vi "ImPro - UI Text.vi"(7 "Directory Path":path, 8 "error in (no error)":errorcluster, 10 "Supervisory Config Cluster Out":T3={"UI Information"={"Header Image"=path "../Data/header.png", "Language"=enum."English", "First Run?"=FALSE, "Setup Camera?"=FALSE, "Device Type"=enum."RCA", "Encoder Type"=enum."Tacho", "Version"=enum."RailMeasurement_CAT", "port"=0, "greyscale"=FALSE, "camera index"=0}, "Test Cluster"={"Operator"="", "Description"="", "Line"="", "Start Position"=450000.0, "Run Length"=31.0, "Sensor A Position"=80000.0, "Rail Side"=FALSE, "Distance Direction"=FALSE, "Path"=path "", "Sensor B Position"=0.0, "Visible Chart Distance"=0.0, "Company"="", "Ref Profile"=""}, "RV-HR Settings Cluster"={"Sensor A Calibration"=0.0, "Integrator Time"=0.0, "Encoder Spacing"=0.0, "Encoder Threshold"=0.0, "Sampling Distance"=0, "Swap Direction?"=FALSE, "Min Walking Speed"=0.0, "Max Walking Speed"=0.0, "Distance Format"=0, "Sensor B Calibration"=0.0, "Tacho Pulses/Rev"=0.0, "Wheel Diameter"=0.0, "Max Short Roughness"=0.0, "Max Long Roughness"=0.0, "Measuring Interval"=0.0, "Measuring Length"=0.0, "Wavelengths"=[], "Device Resolution"=0, "Detect Change in Direction?"=FALSE, "Save Images?"=FALSE, "Image Frequency"=0, "Save Video?"=FALSE, "Image Offset"=0.0, "Start Position at 0m?"=FALSE, "Live Corrug Est.?"=FALSE, "Wavelength Corrug"=0, "Distance Corrug"=0, "Update Corrug"=0}} {"RV-HR Settings Cluster"."Image Frequency" items=["2", "3", "5"]; "RV-HR Settings Cluster"."Device Resolution" items=["0.1 µm", "1 µm", "10 µm"]; "RV-HR Settings Cluster"."Distance Format" items=["kilometres", "miles & chains", "metres", "stations", "miles"]; "RV-HR Settings Cluster"."Sampling Distance" items=["1mm", "2mm"]}, 11 "UI References":T13) -> (0 "error out":errorcluster, 1 "UI Information.Language":T1, 2 "Language Config Cluster Out":T2={"Home"="Home", "Test Setup"="Setup", "Run Test"="Test", "Configure"="Config", "Hardware Viewer"="Viewer", "Review Test"="Review", "Report"="Home", "Exit"="Exit", "Device Connected?"="Device Connected?", "Test in Progress?"="Test in Progress?", "Simulate?"="Simulate?", "Device Type 1"="Corrugation Analysis Trolley", "Device Type 2"="Bi-Corrugation Analysis Trolley", "Device Type 3"="Bi-Corrugation Analysis Trolley", "Device Type 4"="Bi-Corrugation Analysis Trolley", "Device Type 5"="Bi-Corrugation Analysis Trolley", "Device Type 6"="Bi-Corrugation Analysis Trolley", "Device Type 7"="Bi-Corrugation Analysis Trolley", "Software Version"="Version", "Support"="Software by RailMeasurement Limited - Cambridge - UK - support@railmeasurement.com", "Operator"="Operator:", "Test Description"="Description:", "Line"="Description:", "Test Folder Path"="Folder Path:", "Test Folder Path RCA"="Folder Path:", "Start Position"="Start Position:", "Sensor Position"="Sensor Position:", "Sensor A Position"="Sensor A Position:", "Sensor B Position"="Sensor B Position:", "Visible Chart Distance"="Sensor B Position:", "Rail Side"="Rail Side:", "Rail A Side"="Rail A Side:", "Distance Direction"="Distance Direction:", "Start"="Start:", "Distance Travelled"="Distance Travelled:", "Current Position"="Current Position:", "Stop Test"="Stop", "Pause Test"="Save", "Displacement"="Displacement", "Position"="Position", "Sensor Calibration"="Sensor Calibration:", "Sensor A Calibration"="Sensor A Calibration:", "Sensor B Calibration"="Sensor B Calibration:", "Encoder Spacing"="Encoder Spacing:", "Sampling Distance"="Sampling Distance:", "Tacho Pulses/Rev"="Sensor Calibration:", "Wheel Diameter"="Sensor A Calibration:", "Sampling Distances"=["1mm", "2mm"], "Distance Unit"="Distance in:", "Distance Units"=["Kilometres", "miles & chains", "metres", "stations", "miles"], "Swap Direction"="Swap Direction at Run End?", "Language"="Language", "Device Resolution"="Save", "Device Resolutions"=["Kilometres", "miles & chains", "metres", "stations", "miles"], "Detect Change in Direction"="Save", "Save Config"="Save", "Encoder Data"="Encoder Data", "Sensor Data"="Sensor Data", "Sensor A Data"="Sensor A Data", "Sensor B Data"="Sensor B Data", "Voltage"="Voltage", "Time (m:s)"="Time (m:s)", "Unit mm/s/V"="(mm/s)/V", "Unit mm"="mm", "Unit km"="km", "Unit m"="m", "Start Test Message"="m", "Stop Test Message"="km", "Exit Message"="mm", "File Exists Message"="mm", "File Path Invalid Message"="mm", "Combine Error"="mm", "Combine Success"="mm", "Roller Comp Error"="mm", "Test Folder Path (Live)"="mm", "Folder Error"="Sensor B Position:", "Enc Count"="Setup", "Run Start"="mm", "Run End"="mm", "Date"="mm", "Train"="Sensor B Position:", "Location"="Setup", "Notes"="mm", "Heading_1"="mm", "Heading_2"="mm", "Left Rail"="Sensor B Position:", "Right Rail"="Setup", "Left Exclusions"="mm", "Right Exclusions"="mm", "Settings"="mm", "Wavelength Ranges"="Sensor B Position:", "Y-Axis Limits"="Setup", "Exc Limits"="Sensor B Position:", "Other Settings"="Setup", "Distance/Page"="mm", "Distance/Pages"=["Kilometres", "miles & chains", "metres", "stations", "miles"], "Gridlines"="mm", "Report Tolerance"="mm", "Manual Cut"="Sensor B Position:", "Plot Colour"="Distance in:", "Plot Colours"=["Kilometres", "miles & chains", "metres", "stations", "miles"], "EN Standard"="mm", "RiL Standard"="mm", "Custom Standard"="mm", "Resolution"="Distance in:", "Resolutions"=["Kilometres", "miles & chains", "metres", "stations", "miles"], "Exceedence Header"="mm", "Distance (km)"="mm", "Left (%)"="mm", "Right (%)"="Distance in:", "Page"="Distance in:", "Align"="mm", "Main"="mm", "Comparison"="Distance in:", "Offset"="Distance in:", "From"="Distance in:", "To"="Distance in:", "Of"="Distance in:", "File"="mm", "Load New"="mm", "Load Comparison"="Distance in:", "Discard Comparison"="Distance in:", "Print Current Page"="Distance in:", "Print All Pages"="Distance in:", "Print Exceedence Report"="Distance in:", "Plot Main"="Distance in:", "No Comparison Data to Align"="Distance in:", "Run Load Error"="Distance in:", "Report Load Error"="Distance in:", "Cut"="Distance in:", "Remove"="Distance in:", "Config Settings Unsaved"="Distance in:", "Acquisition Paused"="Distance in:", "Please Select One Option Below"="Distance in:", "RCA is Now Stationary"="Distance in:", "Reporting Setting"="Distance in:", "Main Abbreviated"="Distance in:", "Comparison Abbreviated"="Distance in:", "Exceedence Abbreviated"="Distance in:", "Align Comparison"="Distance in:", "Rail Corrugation Analyser Reporting"="Distance in:", "Show Exc. % in Graph"="Distance in:", "Evaluate Sections <100m"="Distance in:", "Evaluate Sections <0.062mile"="Distance in:", "Section Too Short for Evaluation"="Distance in:", "Language Change Prompt"="Distance in:", "Show All"="Distance in:", "Sections_km"="Distance in:", "Sections_mi"="Distance in:", "Vision"="Distance in:", "Vision Report"="Distance in:", "Vision Display"="Distance in:", "Vision Displays"=["Kilometres", "miles & chains", "metres", "stations", "miles"], "Save Images"="Distance in:", "Image Frequency"="Distance in:", "Section"="Distance in:", "Brightness"="Distance in:", "Contrast"="Distance in:", "Shadow"="Distance in:", "Sharpened"="Distance in:", "Apply to all Images"="Distance in:", "Reset"="Distance in:", "Are you sure"="Distance in:", "Image Processing"="Distance in:", "Save Video"="Distance in:", "Image Offset"="Distance in:", "Camera Mode"="Distance in:", "Camera Modes"=["Kilometres", "miles & chains", "metres", "stations", "miles"], "Copy Page"="Distance in:", "Copy Graphs"="Distance in:", "Camera Mode Change Prompt"="Distance in:", "Camera_1 Missing"="Distance in:", "Camera_2 Missing"="Distance in:", "Cameras Missing"="Distance in:", "Camera Setup"="Distance in:", "Camera_1 Connection Error"="Distance in:", "Camera_2 Connection Error"="Distance in:", "Cameras Connection Error"="Distance in:", "No GPS"="Distance in:", "No Signal"="Distance in:", "Camera_1 Connected"="Distance in:", "Camera_1 Not Connected"="Distance in:", "Camera_2 Connected"="Distance in:", "Camera_2 Not Connected"="Distance in:", "Start Position at 0m?"="Distance in:", "Continue"="Distance in:", "New Test, Same Direction"="Distance in:", "New Test, Opposite Direction"="Distance in:", "Stop and Save"="Distance in:", "Live Corrug Estimate"="Distance in:", "Wavelength Corrug"="Distance in:", "Distance Corrug "="Distance in:", "Update Corrug"="Distance in:", "Company"="Distance in:", "Ref Profile "="Distance in:"}, 3 "Support":string)   [LabVIEW 2023]
uses:
  Controls/Language.ctl
  <vilib>/addons/Tools/Unicode/UI Unicode Tools.lvlib
  Controls/Device_Type.ctl
  Controls/UI Init Config Info.ctl
  Controls/Test Cluster.ctl
  Controls/Sampling DIstance.ctl
  Controls/Distance Units.ctl
  Controls/Settings Cluster.ctl
  Controls/Supervisory Config Cluster.ctl
  Controls/Language Text Cluster.ctl
  Controls/EncoderType.ctl
  Controls/Device_Resolution.ctl
  Controls/Software Version.ctl
  Controls/ImPro - UI Refs.ctl
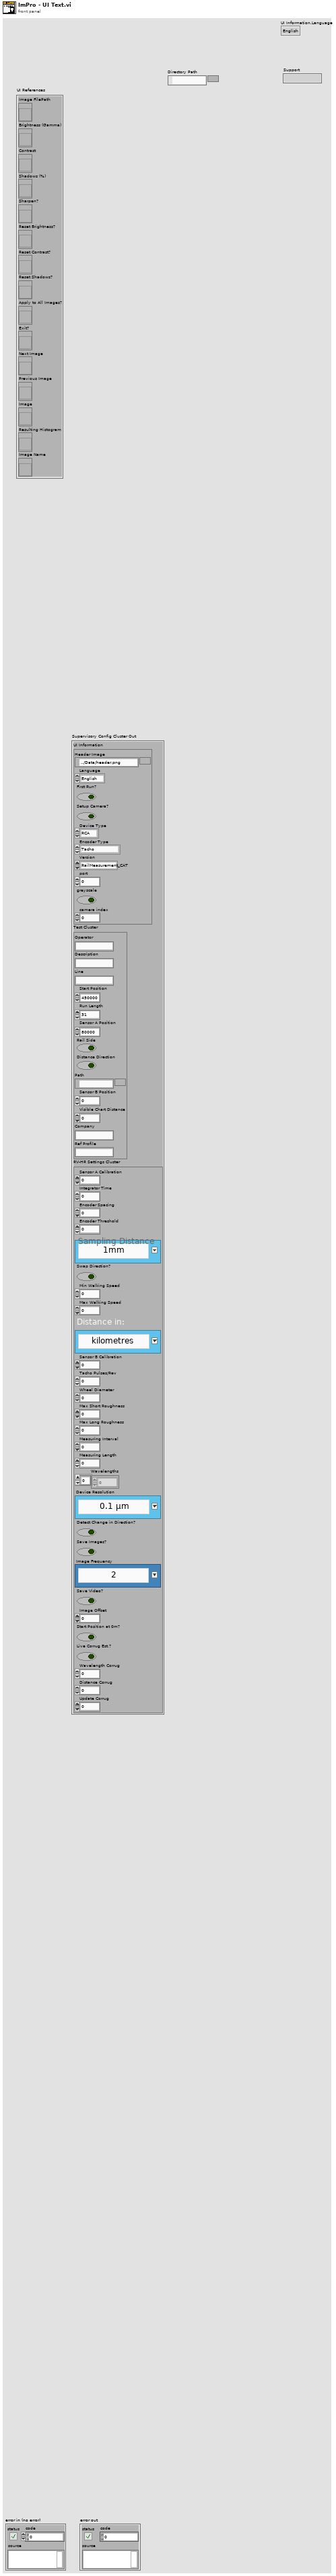
[diagram p1: front panel]
types:
  T1 = typedef "Language.ctl" = enum16{"English", "Chinese", "German"}
  T2 = typedef "Language Text Cluster.ctl" = cluster{"Home":string, "Test Setup":string, "Run Test":string, "Configure":string, "Hardware Viewer":string, "Review Test":string, "Report":string, "Exit":string, "Device Connected?":string, "Test in Progress?":string, "Simulate?":string, "Device Type 1":string, "Device Type 2":string, "Device Type 3":string, "Device Type 4":string, "Device Type 5":string, "Device Type 6":string, "Device Type 7":string, "Software Version":string, "Support":string, "Operator":string, "Test Description":string, "Line":string, "Test Folder Path":string, "Test Folder Path RCA":string, "Start Position":string, "Sensor Position":string, "Sensor A Position":string, "Sensor B Position":string, "Visible Chart Distance":string, "Rail Side":string, "Rail A Side":string, "Distance Direction":string, "Start":string, "Distance Travelled":string, "Current Position":string, "Stop Test":string, "Pause Test":string, "Displacement":string, "Position":string, "Sensor Calibration":string, "Sensor A Calibration":string, "Sensor B Calibration":string, "Encoder Spacing":string, "Sampling Distance":string, "Tacho Pulses/Rev":string, "Wheel Diameter":string, "Sampling Distances":string[], "Distance Unit":string, "Distance Units":string[], "Swap Direction":string, "Language":string, "Device Resolution":string, "Device Resolutions":string[], "Detect Change in Direction":string, "Save Config":string, "Encoder Data":string, "Sensor Data":string, "Sensor A Data":string, "Sensor B Data":string, "Voltage":string, "Time (m:s)":string, "Unit mm/s/V":string, "Unit mm":string, "Unit km":string, "Unit m":string, "Start Test Message":string, "Stop Test Message":string, "Exit Message":string, "File Exists Message":string, "File Path Invalid Message":string, "Combine Error":string, "Combine Success":string, "Roller Comp Error":string, "Test Folder Path (Live)":string, "Folder Error":string, "Enc Count":string, "Run Start":string, "Run End":string, "Date":string, "Train":string, "Location":string, "Notes":string, "Heading_1":string, "Heading_2":string, "Left Rail":string, "Right Rail":string, "Left Exclusions":string, "Right Exclusions":string, "Settings":string, "Wavelength Ranges":string, "Y-Axis Limits":string, "Exc Limits":string, "Other Settings":string, "Distance/Page":string, "Distance/Pages":string[], "Gridlines":string, "Report Tolerance":string, "Manual Cut":string, "Plot Colour":string, "Plot Colours":string[], "EN Standard":string, "RiL Standard":string, "Custom Standard":string, "Resolution":string, "Resolutions":string[], "Exceedence Header":string, "Distance (km)":string, "Left (%)":string, "Right (%)":string, "Page":string, "Align":string, "Main":string, "Comparison":string, "Offset":string, "From":string, "To":string, "Of":string, "File":string, "Load New":string, "Load Comparison":string, "Discard Comparison":string, "Print Current Page":string, "Print All Pages":string, "Print Exceedence Report":string, "Plot Main":string, "No Comparison Data to Align":string, "Run Load Error":string, "Report Load Error":string, "Cut":string, "Remove":string, "Config Settings Unsaved":string, "Acquisition Paused":string, "Please Select One Option Below":string, "RCA is Now Stationary":string, "Reporting Setting":string, "Main Abbreviated":string, "Comparison Abbreviated":string, "Exceedence Abbreviated":string, "Align Comparison":string, "Rail Corrugation Analyser Reporting":string, "Show Exc. % in Graph":string, "Evaluate Sections <100m":string, "Evaluate Sections <0.062mile":string, "Section Too Short for Evaluation":string, "Language Change Prompt":string, "Show All":string, "Sections_km":string, "Sections_mi":string, "Vision":string, "Vision Report":string, "Vision Display":string, "Vision Displays":string[], "Save Images":string, "Image Frequency":string, "Section":string, "Brightness":string, "Contrast":string, "Shadow":string, "Sharpened":string, "Apply to all Images":string, "Reset":string, "Are you sure":string, "Image Processing":string, "Save Video":string, "Image Offset":string, "Camera Mode":string, "Camera Modes":string[], "Copy Page":string, "Copy Graphs":string, "Camera Mode Change Prompt":string, "Camera_1 Missing":string, "Camera_2 Missing":string, "Cameras Missing":string, "Camera Setup":string, "Camera_1 Connection Error":string, "Camera_2 Connection Error":string, "Cameras Connection Error":string, "No GPS":string, "No Signal":string, "Camera_1 Connected":string, "Camera_1 Not Connected":string, "Camera_2 Connected":string, "Camera_2 Not Connected":string, "Start Position at 0m?":string, "Continue":string, "New Test, Same Direction":string, "New Test, Opposite Direction":string, "Stop and Save":string, "Live Corrug Estimate":string, "Wavelength Corrug":string, "Distance Corrug ":string, "Update Corrug":string, "Company":string, "Ref Profile ":string}
  T3 = typedef "Supervisory Config Cluster.ctl" = cluster{"UI Information":T4, "Test Cluster":T8, "RV-HR Settings Cluster":T9}
  T4 = typedef "UI Init Config Info.ctl" = cluster{"Header Image":path, "Language":T1, "First Run?":bool, "Setup Camera?":bool, "Device Type":T5, "Encoder Type":T6, "Version":T7, "port":i32, "greyscale":bool, "camera index":i32}
  T5 = typedef "Device_Type.ctl" = enum16{"CAT", "Bi-CAT", "YRCA", "RCA", "RV-HR", "TV-HR"}
  T6 = typedef "EncoderType.ctl" = enum16{"Tacho", "Quadrature"}
  T7 = typedef "Software Version.ctl" = enum16{"RailMeasurement_CAT", "RailMeasurement_Master", "RailMeasurement_RCA", "RailMeasurement_CAT-V", "RailMeasurement_RCA-V", "RailMeasurement_RV-HR"}
  T8 = typedef "Test Cluster.ctl" = cluster{"Operator":string, "Description":string, "Line":string, "Start Position":dbl, "Run Length":dbl, "Sensor A Position":dbl, "Rail Side":bool, "Distance Direction":bool, "Path":path, "Sensor B Position":dbl, "Visible Chart Distance":dbl, "Company":string, "Ref Profile":string}
  T9 = typedef "Settings Cluster.ctl" = cluster{"Sensor A Calibration":dbl, "Integrator Time":dbl, "Encoder Spacing":dbl, "Encoder Threshold":dbl, "Sampling Distance":T10, "Swap Direction?":bool, "Min Walking Speed":dbl, "Max Walking Speed":dbl, "Distance Format":T11, "Sensor B Calibration":dbl, "Tacho Pulses/Rev":dbl, "Wheel Diameter":dbl, "Max Short Roughness":dbl, "Max Long Roughness":dbl, "Measuring Interval":dbl, "Measuring Length":dbl, "Wavelengths":dbl[], "Device Resolution":T12, "Detect Change in Direction?":bool, "Save Images?":bool, "Image Frequency":T10, "Save Video?":bool, "Image Offset":dbl, "Start Position at 0m?":bool, "Live Corrug Est.?":bool, "Wavelength Corrug":u8, "Distance Corrug":u8, "Update Corrug":u8}
  T10 = typedef "Sampling DIstance.ctl" = u16
  T11 = typedef "Distance Units.ctl" = u16
  T12 = typedef "Device_Resolution.ctl" = u16
  T13 = typedef "ImPro - UI Refs.ctl" = cluster{"Image FilePath":refnum<vi>, "Brightness (Gamma)":refnum<vi>, "Contrast":refnum<vi>, "Shadows (%)":refnum<vi>, "Sharpen?":refnum<vi>, "Reset Brightness?":refnum<vi>, "Reset Contrast?":refnum<vi>, "Reset Shadows?":refnum<vi>, "Apply to All Images?":refnum<vi>, "Exit?":refnum<vi>, "Next Image":refnum<vi>, "Previous Image":refnum<vi>, "Image":refnum<vi>, "Resulting Histogram":refnum<vi>, "Image Name":refnum<vi>}
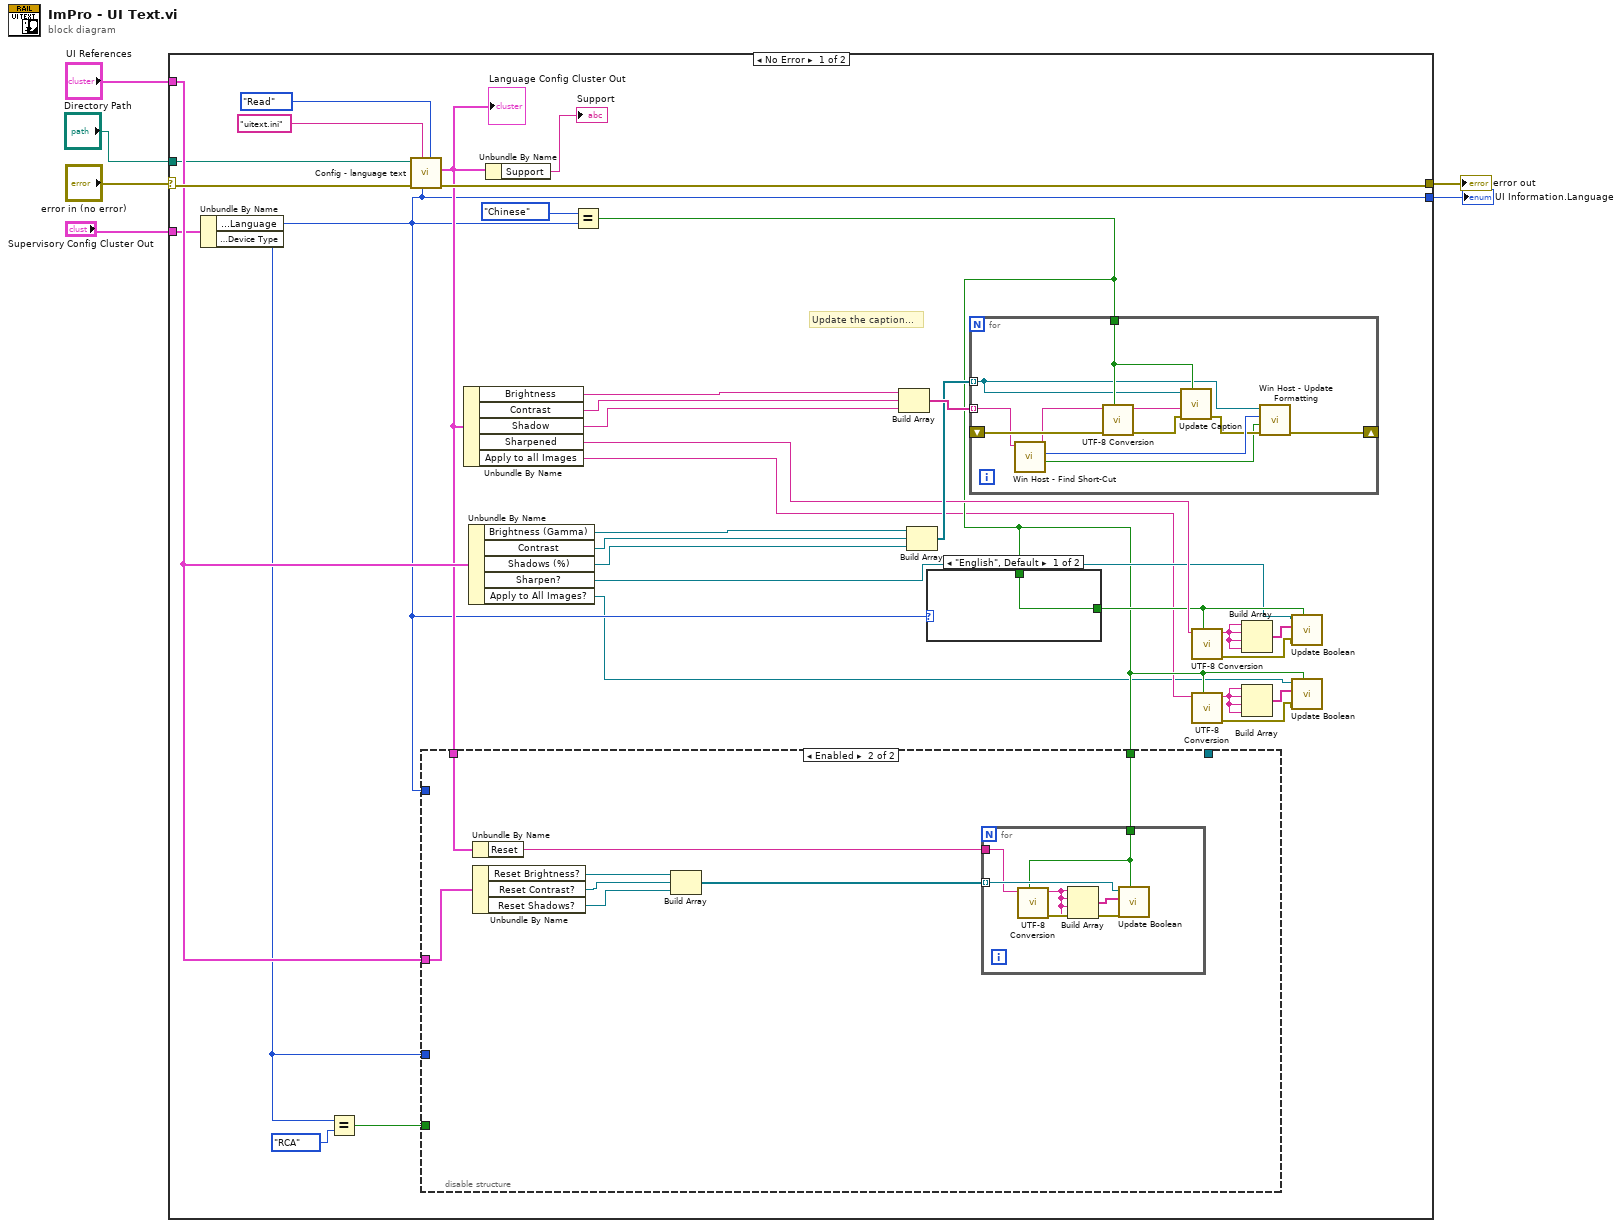
[diagram p0: block diagram]
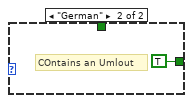
[diagram p2: hidden frame]
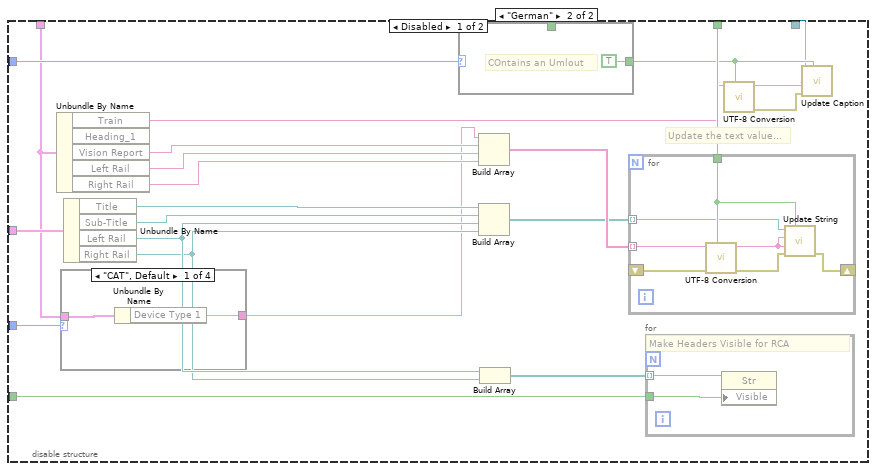
[diagram p3: hidden frame]
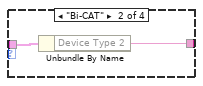
[diagram p4: hidden frame]
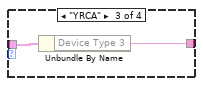
[diagram p5: hidden frame]
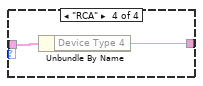
[diagram p6: hidden frame]
diagram:
  n1 = case shown="No Error" "error in (no error)" {
    selector: "error in (no error)" -> [w40 w109]
    tunnel: [w39 w109] -> w5
    tunnel: "UI References" -> [w34 _]
    tunnel: "Supervisory Config Cluster Out" -> [w32 _]
    tunnel: "Directory Path" -> [w33 _]
    tunnel: [w18 _] -> w1
    frame No Error {
      # "Update the caption..."
      n2 = Unbundle By Name(w32) -> ("UI Information.Language"=w18:T1, "UI Information.Device Type"=w23:T5)
      n3 = Equal?(x=w23, y=Device_Type."RCA") -> (x = y?=w24:bool)
      n4 = call "Config - language text.vi"(".ini Controller"=enum16{"Read", "Write"}."Read", "Language"=w18, ".ini filename"="uitext.ini", "error in (no error)"=w40, "Directory Path"=w33) -> ("error out"=w39:errorcluster, "Language Config Cluster Out"=w22:T2)  [unwired: 4 in, 1 out]
      "Language Config Cluster Out" <- w22
      n5 = Unbundle By Name(w22) -> ("Brightness"=w26:string, "Contrast"=w21:string, "Shadow"=w20:string, "Sharpened"=w19:string, "Apply to all Images"=w8:string)
      n6 = Unbundle By Name(w34) -> ("Brightness (Gamma)"=w29:refnum<vi>, "Contrast"=w28:refnum<vi>, "Shadows (%)"=w27:refnum<vi>, "Sharpen?"=w15:refnum<vi>, "Apply to All Images?"=w7:refnum<vi>)
      n7 = Unbundle By Name(w22) -> ("Support"=→"Support":string)
      n8 = Equal?(x=Language."Chinese" ("UI Information.Language"), y=w18) -> (x = y?=w9:bool)
      n9 = disable-structure shown="Enabled" {
        disable-tunnel: w34 -> [w64 w90]
        disable-tunnel: w9 -> [w63 w91]
        disable-tunnel: w18 -> [w62 _]
        disable-tunnel: _ -> [w51 _]
        disable-tunnel: w24 -> [w46 _]
        disable-tunnel: w23 -> [w45 _]
        disable-tunnel: w22 -> [w44 w85]
        frame Disabled {
          # "Update the text value..."
          n10 = Unbundle By Name(w44) -> ("Train"=w50:string, "Vision Report"=w55:string, "Left Rail"=w56:string, "Right Rail"=w57:string)  [unwired: 1 out]
          n11 = case shown="\"CAT\", Default" w45 {
            tunnel: w44 -> [w66 w68 w70 w72]
            tunnel: [w65 w67 w69 w71] -> w43
            frame "CAT", Default {
              n12 = Unbundle By Name(w66) -> ("Device Type 1"=w65:string)
            }
            frame "Bi-CAT" {
              n13 = Unbundle By Name(w68) -> ("Device Type 2"=w67:string)
            }
            frame "YRCA" {
              n14 = Unbundle By Name(w70) -> ("Device Type 3"=w69:string)
            }
            frame "RCA" {
              n15 = Unbundle By Name(w72) -> ("Device Type 4"=w71:string)
            }
          }
          n16 = Unbundle By Name(w64) -> ("Title"=w58:refnum<vi>, "Sub-Title"=w59:refnum<vi>, "Left Rail"=w49:refnum<vi>, "Right Rail"=w48:refnum<vi>)
          n17 = case shown="\"German\"" w62 {
            tunnel: w63 -> [w73 _]
            tunnel: [w73 TRUE] -> w52
            frame "English", Default {
            }
            frame "German" {
              # "COntains an Umlout"
            }
          }
          n18 = Build Array(w43, w55, w56, w57) -> (w61:string[])
          n19 = Build Array(w58, w59, w49, w48) -> (w60:refnum<vi>[])
          n20 = Build Array(w49, w48) -> (w47:refnum<vi>[])
          n21 = for {
            tunnel: w61 -> [w78] mode=indexing
            tunnel: w63 -> [w80]
            tunnel: w60 -> [w79] mode=indexing
            shift-right: [w81] -> _
            shift-left: _ -> [w83]
            n22 = call "UTF-8 Conversion.vi"("Unicode?"=w80, "error in"=w83, "Config String"=w78) -> ("error out"=w82:errorcluster, "Unicode/ANSI string"=w77:string)  [unwired: 7 in]
            n23 = call <vilib>:"Update String.vi"("Interpret as Unicode (T)"=w80, "error in (no error)"=w82, "Caption"=w77, "String Value"=w77, "String Control Reference"=w79) -> ("error out"=w81:errorcluster)  [unwired: 3 in, 1 out]
          }
          n24 = for {
            tunnel: w47 -> [w76] mode=indexing
            tunnel: w46 -> [w75]
            # "Make Headers Visible for RCA"
            n25 = property class="Str"(reference=w76, "Visible"=w75) -> ()  [unwired: 1 in, 2 out]
          }
          n26 = call "UTF-8 Conversion.vi"("Unicode?"=w52, "Config String"=w50) -> ("error out"=w54:errorcluster, "Unicode/ANSI string"=w53:string)  [unwired: 8 in]
          n27 = call <vilib>:"Update Caption.vi"("Interpret as Unicode (T)"=w52, "error in (no error)"=w54, "Caption"=w53, "Control Reference"=w51) -> ()  [unwired: 4 in, 2 out]
        }
        frame Enabled {
          n28 = Unbundle By Name(w85) -> ("Reset"=w84:string)
          n29 = Unbundle By Name(w90) -> ("Reset Brightness?"=w89:refnum<vi>, "Reset Contrast?"=w88:refnum<vi>, "Reset Shadows?"=w87:refnum<vi>)
          n30 = Build Array(w89, w88, w87) -> (w86:refnum<vi>[])
          n31 = for {
            tunnel: w91 -> [w95]
            tunnel: w86 -> [w96] mode=indexing
            tunnel: w84 -> [w92]
            n32 = call "UTF-8 Conversion.vi"("Unicode?"=w95, "Config String"=w92) -> ("error out"=w97:errorcluster, "Unicode/ANSI string"=w94:string)  [unwired: 8 in]
            n33 = Build Array(w94, w94, w94, w94) -> (w93:string[])
            n34 = call <vilib>:"Update Boolean.vi"("Interpret as Unicode (T)"=w95, "error in (no error)"=w97, "Boolean Texts [4]"=w93, "Boolean Reference"=w96) -> ()  [unwired: 4 in, 2 out]
          }
        }
      }
      n35 = Build Array(w26, w21, w20) -> (w31:string[])
      n36 = Build Array(w29, w28, w27) -> (w30:refnum<vi>[])
      n37 = case shown="\"English\", Default" w18 {
        tunnel: w9 -> [w41 _]
        tunnel: [w41 TRUE] -> w16
        frame "English", Default {
        }
        frame "German" {
          # "COntains an Umlout"
        }
      }
      n38 = for {
        tunnel: w31 -> [w104] mode=indexing
        tunnel: w9 -> [w107]
        tunnel: w30 -> [w101] mode=indexing
        shift-right: [w99] -> _
        shift-left: _ -> [w105]
        n39 = call "Win Host - Find Short-Cut.vi"("Language in"=w104) -> ("Short-Cut?"=w98:bool, "S/CUT Index"=w102:i32, "Language out"=w103:string)  [unwired: 8 in]
        n40 = call "UTF-8 Conversion.vi"("Unicode?"=w107, "error in"=w105, "Config String"=w103) -> ("error out"=w106:errorcluster, "Unicode/ANSI string"=w108:string)  [unwired: 7 in]
        n41 = call <vilib>:"Update Caption.vi"("Interpret as Unicode (T)"=w107, "error in (no error)"=w106, "Caption"=w108, "Control Reference"=w101) -> ("error out"=w100:errorcluster)  [unwired: 4 in, 1 out]
        n42 = call "Win Host - Update Formatting.vi"("error in (no error)"=w100, "Short-Cut?"=w98, "Index"=w102, "Control in"=w101) -> ("error out"=w99:errorcluster)  [unwired: 7 in]
      }
      n43 = call "UTF-8 Conversion.vi"("Unicode?"=w16, "Config String"=w19) -> ("error out"=w17:errorcluster, "Unicode/ANSI string"=w13:string)  [unwired: 8 in]
      n44 = call "UTF-8 Conversion.vi"("Unicode?"=w9, "Config String"=w8) -> ("error out"=w10:errorcluster, "Unicode/ANSI string"=w12:string)  [unwired: 8 in]
      n45 = Build Array(w13, w13, w13, w13) -> (w14:string[])
      n46 = Build Array(w12, w12, w12, w12) -> (w11:string[])
      n47 = call <vilib>:"Update Boolean.vi"("Interpret as Unicode (T)"=w16, "error in (no error)"=w17, "Boolean Texts [4]"=w14, "Boolean Reference"=w15) -> ()  [unwired: 4 in, 2 out]
      n48 = call <vilib>:"Update Boolean.vi"("Interpret as Unicode (T)"=w9, "error in (no error)"=w10, "Boolean Texts [4]"=w11, "Boolean Reference"=w7) -> ()  [unwired: 4 in, 2 out]
    }
    frame Error {
    }
  }
  "error out" <- w5
  "UI Information.Language" <- w1
